vi "ROI group-Extract group names from setup array.vi"(1 "Groups setup":T1[](array[typedef]) {"Group region specifier cluster"."Contours"."Type" items=["No Selection", "Point", "Line", "Rectangle", "Oval", "Polygon", "Freehand Region", "Annulus", "Unused2", "Unused3", "Broken Line", "Freehand Line", "Rotated Rectangle"]}) -> (0 "Group Names Array":string[](array[string]))   [LabVIEW 2013]
uses:
  ROI Selection Interface/ROI group info cluster.ctl
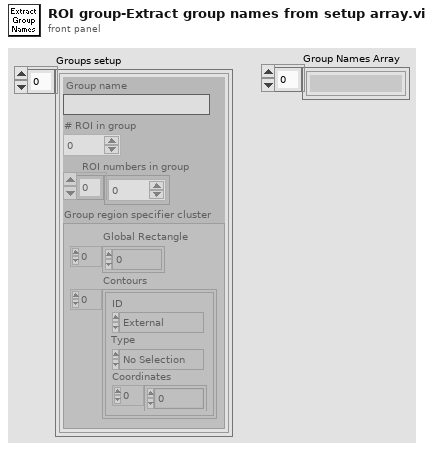
[diagram p1: front panel]
types:
  T1 = typedef "ROI group info cluster.ctl" = cluster{"Group name":string, "# ROI in group":i32, "ROI numbers in group":i32[], "Group region specifier cluster":T2}
  T2 = typedef "ROI Descriptor" = cluster{"Global Rectangle":i32[], "Contours":cluster{"ID":enum32{"External", "Internal"}, "Type":u32, "Coordinates":i32[]}[]}
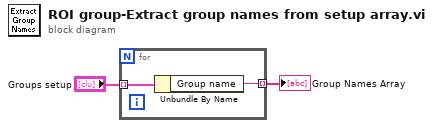
[diagram p0: block diagram]
diagram:
  n1 = for {
    tunnel: "Groups setup" -> [w4] mode=indexing
    tunnel: [w3] -> w2 mode=indexing
    n2 = Unbundle By Name(w4) -> ("Group name"=w3:string)
  }
  "Group Names Array" <- w2
